vi "create_black_screen.vi"() -> (1 "img_black_screen":T1(plugin-control))   [LabVIEW 2011]
uses:
  global_vars.vi
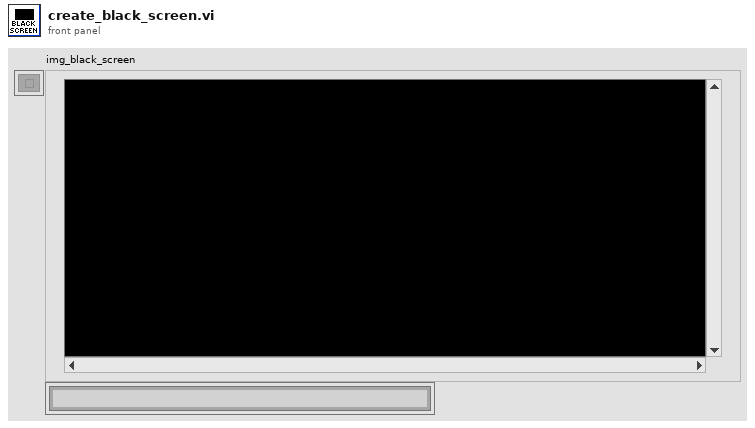
[diagram p1: front panel]
types:
  T1 = typedef "IMAQ Image.ctl" = refnum<image>
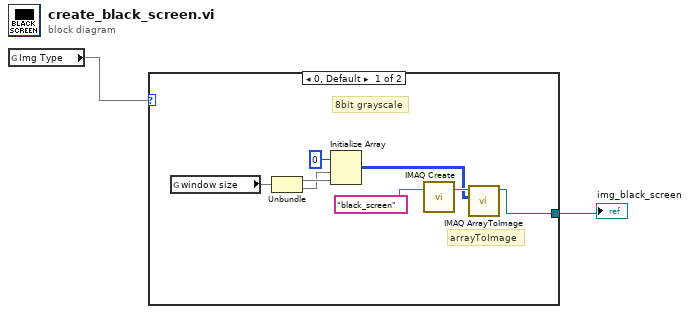
[diagram p0: block diagram]
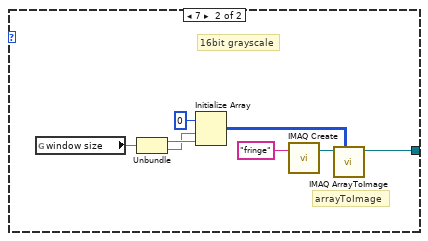
[diagram p2: hidden frame]
diagram:
  n1 = global read "global_vars.vi" "Img Type"() -> (w2)
  n2 = case shown="0, Default" w2 {
    tunnel: [w3 w12] -> w1
    frame 0, Default {
      # "8bit grayscale"
      # "arrayToImage"
      n3 = global read "global_vars.vi" "window size"() -> (w6)
      n4 = Unbundle(w6) -> (w10, w9)
      n5 = Initialize Array(u8 0 ("element"), w9, w10) -> (w4:u8[][])
      n6 = call "IMAQ Create"("Image Name"="black_screen") -> ("New Image"=w8:T1)  [unwired: 3 in, 2 out]
      n7 = call "IMAQ ArrayToImage"("Image Pixels (U8)"=w4, "Image"=w8) -> ("Image Out"=w3:T1)  [unwired: 8 in, 1 out]
    }
    frame 7 {
      # "16bit grayscale"
      # "arrayToImage"
      n8 = global read "global_vars.vi" "window size"() -> (w14)
      n9 = Unbundle(w14) -> (w18, w17)
      n10 = Initialize Array(u16 0 ("element"), w17, w18) -> (w11:u16[][])
      n11 = call "IMAQ Create"("Image Name"="fringe") -> ("New Image"=w16:T1)  [unwired: 3 in, 2 out]
      n12 = call "IMAQ ArrayToImage"("Image Pixels (U16)"=w11, "Image"=w16) -> ("Image Out"=w12:T1)  [unwired: 8 in, 1 out]
    }
  }
  "img_black_screen" <- w1
